vi "Compare_pyWebscraper_Data.vi"(8 "error in (no error)":errorcluster, 10 "Expected String":string, 11 "Input Result":string) -> (0 "error out":errorcluster, 3 "Pass?":bool)   [LabVIEW 2025]
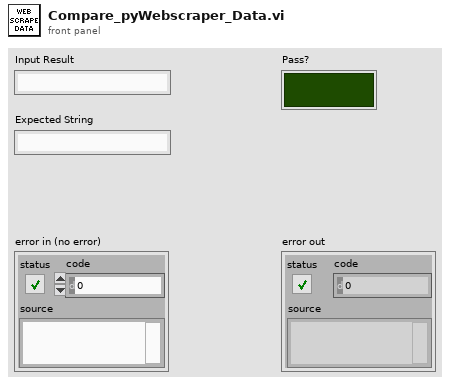
[diagram p1: front panel]
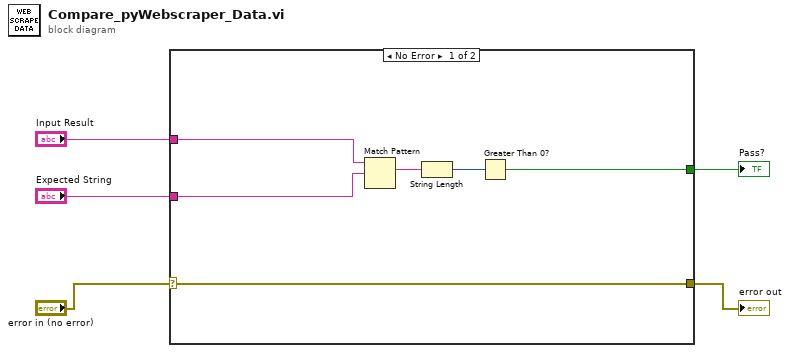
[diagram p0: block diagram]
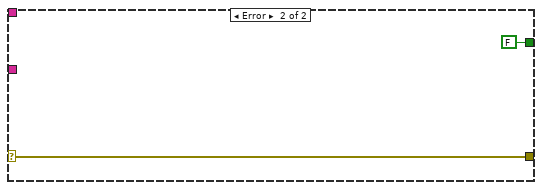
[diagram p2: hidden frame]
diagram:
  n1 = case shown="No Error" "error in (no error)" {
    selector: "error in (no error)" -> [w6 w13]
    tunnel: [w6 w13] -> w4
    tunnel: "Input Result" -> [w11 _]
    tunnel: "Expected String" -> [w10 _]
    tunnel: [w7 FALSE] -> w1
    frame No Error {
      n2 = Match Pattern(string=w11, regular expression=w10) -> (match substring=w9:string)  [unwired: 1 in, 3 out]
      n3 = String Length(string=w9) -> (length=w8:i32)
      n4 = Greater Than 0?(x=w8) -> (x > 0?=w7:bool)
    }
    frame Error {
    }
  }
  "error out" <- w4
  "Pass?" <- w1
